vi "nominal dataset update begin.vi"(8 "error in (no error)":errorcluster, 11 "out_staging":i32) -> (0 "error out":errorcluster, 2 "function return":i32, 3 "out_staging out":i32)   [LabVIEW 2020, in "client.lvlib"]
doc: "int32_t nominal_dataset_update_begin(int32_t *out_staging);"
uses:
  client.lvlib
  nominalClient_64.dll
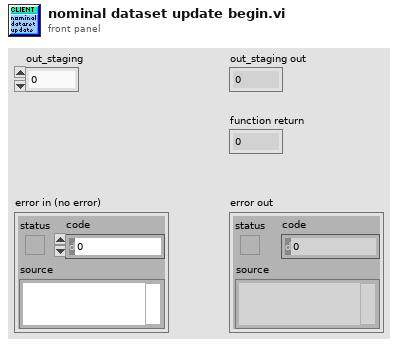
[diagram p1: front panel]
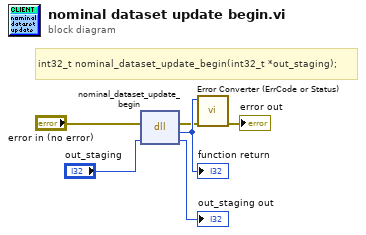
[diagram p0: block diagram]
diagram:
  # "int32_t nominal_dataset_update_begin(int32_t *out_staging);"
  n1 = dll-call lib="C:/code/labview-client-rs/lv_src/client/nominalClient_64.*" fn="nominal_dataset_update_begin"(error in="error in (no error)", "out_staging"="out_staging") -> (error out=w2:errorcluster, w6:i32, "out_staging"=→"out_staging out":i32)  [unwired: 2 in, 1 out]
  "function return" <- w6
  n2 = call "Error Converter (ErrCode or Status).vi"("error in (no error)"=w2, "error code"=w6) -> ("error out"=→"error out":errorcluster)  [unwired: 9 in]
